vi "Stop Communication.vi"(8 "error in (no error)":errorcluster, 11 "Serial Communication in":refnum<class "Serial Communication.lvclass">) -> (0 "error out":errorcluster, 3 "Serial Communication out":refnum<class "Serial Communication.lvclass">)   [LabVIEW 2018, in "Serial Communication.lvclass"]
uses:
  Serial Communication.lvclass
  Serial Communication.lvclass/Serial Communication.ctl
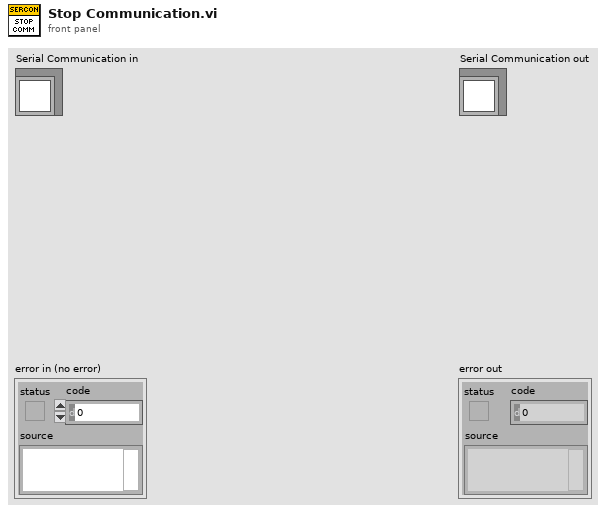
[diagram p1: front panel]
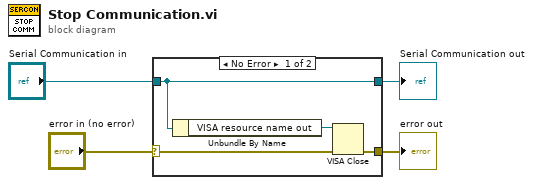
[diagram p0: block diagram]
diagram:
  n1 = case shown="No Error" "error in (no error)" {
    selector: "error in (no error)" -> [w8 w10]
    tunnel: [w7 w10] -> w2
    tunnel: [w6 w9] -> w1
    tunnel: "Serial Communication in" -> [w6 w9]
    frame No Error {
      n2 = Unbundle By Name(w6) -> ("VISA resource name out"=w5:refnum<visa-resource-name>)
      n3 = VISA Close(VISA resource name=w5, error in (no error)=w8) -> (error out=w7:errorcluster)
    }
    frame Error {
    }
  }
  "error out" <- w2
  "Serial Communication out" <- w1
